vi "LAESI_MSI.vi"() -> ()   [LabVIEW 2016]
uses:
  Utility/Global Constants.vi
  Utility/Global_Laser.vi
panel:
  in  "Ceiling":sgl=6.0
  out "Count":u32
  out "LCount":u32
  out "#Stps Y-Axis":i32
  out "#Stps X-Axis":i32
  out "All done":bool
  in  "Offset Z-Axis":sgl=6.3
  in  "Abort!":bool
  out "Abort in Progress":bool
  out "Status?":bool
  out "Current X-Position":i32
  out "Current Y-Position":i32
  in  "ProFile Path":path=path "C:/Users/msg-synapt/Documents/Doktorat/ProFileCSVs/2019/test.csv"
  in  "Energy":i16(slide)=100 min=0 max=100 step=1 scale=0.0..100.0
  in  "#Pulses":string="15"
  in  "Step Size in mm":sgl=0.1
  in  "Y-Axis":sgl=1.0
  in  "Offset Y-Axis":sgl=2.0
  in  "X-Axis":sgl=1.0
  in  "Offset X-Axis":sgl=10.0
  in  "B-Axis":refnum<k7>(container)
  in  "Z-Axis":refnum<k7>(container)
  in  "Y-Axis":refnum<k7>(container)
  in  "X-Axis":refnum<k7>(container)
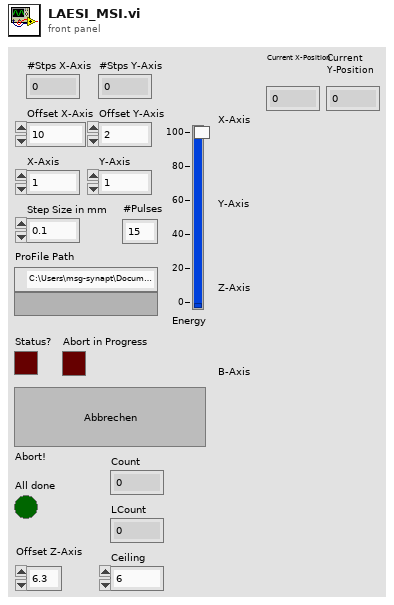
[diagram p1: front panel]
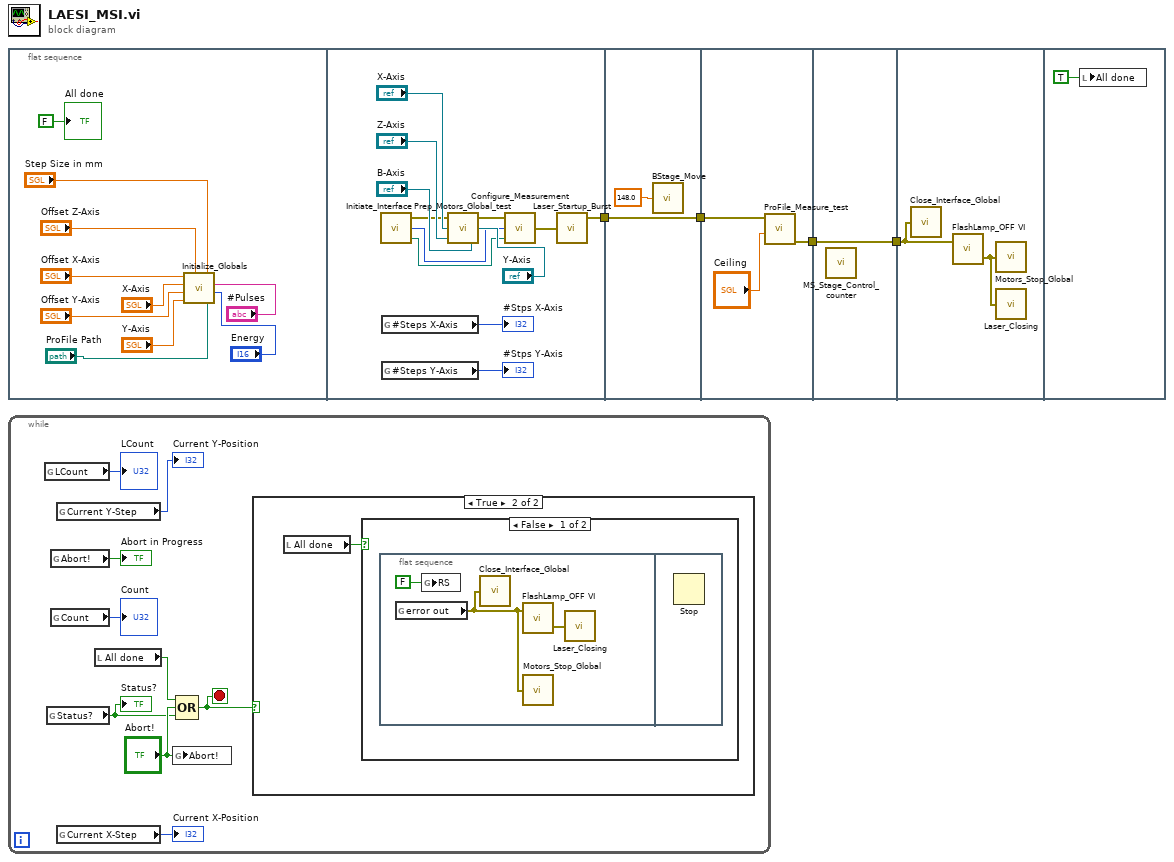
[diagram p0: block diagram]
diagram:
  n1 = flat-sequence {
    tunnel: [w17] -> w2
    tunnel: w2 -> [w28]
    tunnel: [w28] -> w1
    tunnel: w1 -> [w31]
    tunnel: [w30] -> w3
    tunnel: [w32] -> w4
    tunnel: w3 -> [w32]
    tunnel: w4 -> [w34]
    frame #0 {
      n2 = call "Initialize_Globals.vi"("ProFile Path"="ProFile Path", "Energy"="Energy", "#Pulses"="#Pulses", "Step Size in mm"="Step Size in mm", "Offset Z-Axis"="Offset Z-Axis", "Y-Axis"="Y-Axis", "Offset Y-Axis"="Offset Y-Axis", "X-Axis"="X-Axis", "Offset X-Axis"="Offset X-Axis") -> ()
      "All done" <- FALSE ("All done")
    }
    frame #1 {
      n3 = call "Initiate_Interface.vi"() -> ("DLL-Path"=w19:path, "instanceHandle"=w20:u32, "Fehler (Ausgang)"=w22:errorcluster)
      n4 = global read "Global Constants.vi" "#Steps X-Axis"() -> (→"#Stps X-Axis":i32)
      n5 = global read "Global Constants.vi" "#Steps Y-Axis"() -> (→"#Stps Y-Axis":i32)
      n6 = call "Prep_Motors_Global_test.vi"("B-Axis"="B-Axis", "Y-Axis"="Y-Axis", "Z-Axis"="Z-Axis", "X-Axis"="X-Axis", "Error In"=w22) -> ("Error Out"=w21:errorcluster)
      n7 = call "Configure_Measurement.vi"("DLL-Path"=w19, "instanceHandle"=w20, "Error In"=w21) -> ("Fehler (Ausgang)"=w18:errorcluster)
      n8 = call "Laser_Startup_Burst.vi"("Error In"=w18) -> ("Error Out"=w17:errorcluster)  [unwired: 1 out]
    }
    frame #2 {
      n9 = call "BStage_Move.vi"("Position"=sgl 148.0) -> ()
    }
    frame #3 {
      n10 = call "ProFile_Measure_test.vi"("Ceiling"="Ceiling", "error in"=w31) -> ("error out"=w30:errorcluster)  [unwired: 1 in]
    }
    frame #4 {
      n11 = call "MS_Stage_Control_counter.vi"() -> ()  [unwired: 12 in]
    }
    frame #5 {
      n12 = call "Close_Interface_Global.vi"("Error In"=w34) -> ()
      n13 = call "FlashLamp_OFF VI.vi"("Error In"=w34) -> ("error out"=w33:errorcluster)
      n14 = call "Motors_Stop_Global.vi"("error in"=w33) -> ()
      n15 = call "Laser_Closing.vi"("Error In"=w33) -> ()
    }
    frame #6 {
      n16 = local write "All done"(TRUE) -> ()
    }
  }
  n17 = while {
    stop <- w43 stop-if-true
    n18 = global read "Global_Laser.vi" "LCount"() -> (→"LCount":u32)
    n19 = global read "Global Constants.vi" "Status?"() -> (w41:bool)
    "Status?" <- w41
    n20 = global read "Global Constants.vi" "Abort!"() -> (→"Abort in Progress":bool)
    n21 = global read "Global Constants.vi" "Count"() -> (→"Count":u32)
    n22 = global read "Global Constants.vi" "Current Y-Step"() -> (→"Current Y-Position":i32)
    n23 = global read "Global Constants.vi" "Current X-Step"() -> (→"Current X-Position":i32)
    n24 = local read "All done"() -> (w38:bool)
    n25 = global write "Global Constants.vi" "Abort!"("Abort!") -> ()
    n26 = Compound Arithmetic op=OR(w38, "Abort!", w41) -> (w43:bool)
    n27 = case shown="True" w43 {
      frame False {
      }
      frame True {
        n28 = local read "All done"() -> (w45:bool)
        n29 = case shown="False" w45 {
          frame False {
            n30 = flat-sequence {
              frame #0 {
                n31 = global read "Global Constants.vi" "error out"() -> (w46:errorcluster)
                n32 = global write "Global Constants.vi" "RS"(FALSE) -> ()
                n33 = call "Close_Interface_Global.vi"("Error In"=w46) -> ()
                n34 = call "FlashLamp_OFF VI.vi"("Error In"=w46) -> ("error out"=w47:errorcluster)
                n35 = call "Motors_Stop_Global.vi"("error in"=w46) -> ()
                n36 = call "Laser_Closing.vi"("Error In"=w47) -> ()
              }
              frame #1 {
                n37 = Stop() -> ()  [unwired: 1 in]
              }
            }
          }
          frame True {
          }
        }
      }
    }
  }
